vi "Read Stimulus Array.vi"(7 "Channel (1)":i32=1, 8 "error in (no error)":errorcluster, 11 "VISA resource name":refnum<visa-resource-name>) -> (0 "error out":errorcluster, 2 "Stimulus Data":dbl[](array[numeric]), 3 "VISA resource name out":refnum<visa-resource-name>)   [LabVIEW 2011, in "Agilent ENA Series.lvlib"]
doc: "For selected channel, reads out the frequencies of all measurement point."
uses:
  Agilent ENA Series.lvlib
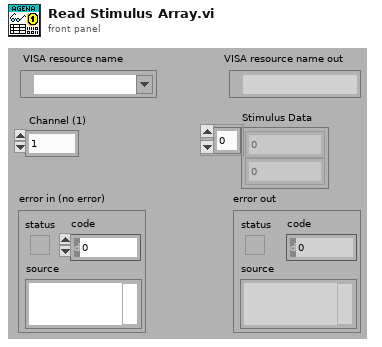
[diagram p1: front panel]
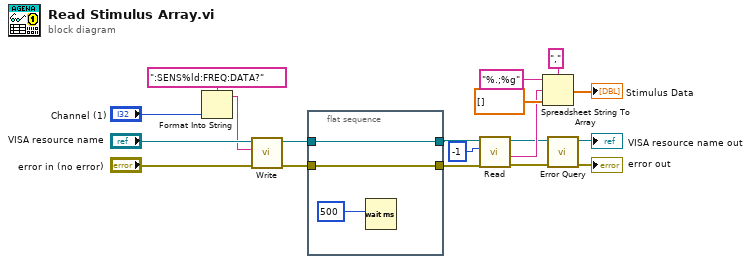
[diagram p0: block diagram]
diagram:
  n1 = Format Into String(format string=":SENS%ld:FREQ:DATA?", "Channel (1)") -> (resulting string=w15:string)  [unwired: 2 in, 1 out]
  n2 = call "Write.vi"("error in (no error)"="error in (no error)", "String ()"=w15, "VISA resource name"="VISA resource name") -> ("error out"=w7:errorcluster, "VISA resource name out"=w8:refnum<visa-resource-name>)  [unwired: 6 in, 1 out]
  n3 = flat-sequence {
    tunnel: w8 -> [w20]
    tunnel: w7 -> [w22]
    tunnel: [w22] -> w5
    tunnel: [w20] -> w6
    frame #0 {
      n4 = Wait (ms)(milliseconds to wait=500) -> ()  [unwired: 1 out]
    }
  }
  n5 = call "Read.vi"("error in (no error)"=w5, "Number Of Bytes"=-1, "VISA resource name"=w6) -> ("error out"=w2:errorcluster, "String"=w11:string, "VISA resource name out"=w4:refnum<visa-resource-name>)  [unwired: 5 in, 1 out]
  n6 = Spreadsheet String To Array(delimiter (Tab)=",", format string="%.;%g", spreadsheet string=w11, array type (2D Dbl)=dbl[] []) -> (array=→"Stimulus Data":dbl[])
  n7 = call "Error Query.vi"("error in (no error)"=w2, "VISA resource name"=w4) -> ("error out"=→"error out":errorcluster, "VISA resource name out"=→"VISA resource name out":refnum<visa-resource-name>)  [unwired: 6 in, 2 out]
